vi "Init User Prompt.vi"(0 "Custom Device Ref in":T2 format="%.0x", 11 "error in":errorcluster) -> (3 "Physical Device Name":string, 4 "Temperature Units":T1 items=["Celcius", "Fahrenheit", "Kelvin", "Rankine"], 6 "Dev Chan Count":u32, 8 "High Side Resistor":dbl, 10 "Low Side Resistor":dbl, 15 "error out":errorcluster)   [LabVIEW 2011, in "Simulated Thermocouple Custom Device.lvlib"]
uses:
  Simulated Thermocouple Custom Device.lvlib
  <vilib>/NI Veristand/Custom Device API/Custom Device Item Ref.ctl
  TC Unit Selector.ctl
  Device Settings.ctl
  <vilib>/NI Veristand/Custom Device API/Get Item Property (Variant).vi
  <vilib>/NI Veristand/Custom Device API/Custom Device API.lvlib
panel:
  in  "Device Channel Count":u16(ring)=6 items=["2", "4", "8", "12", "16", "24", "32"]
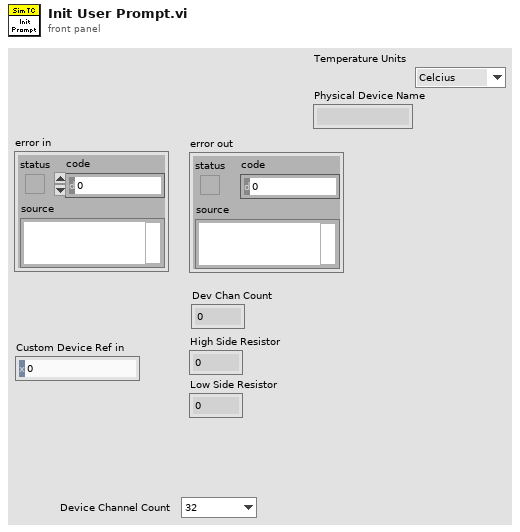
[diagram p1: front panel]
types:
  T1 = typedef "Simulated Thermocouple Custom Device.lvlib/TC Unit Selector.ctl" = u16
  T2 = typedef "Custom Device API.lvlib/Custom Device Item Ref.ctl" = u64
  T3 = typedef "Simulated Thermocouple Custom Device.lvlib/Device Settings.ctl" = cluster{"High Side Resistance (Ohms)":dbl, "Low Side Resistance (Ohms)":dbl, "Temperature Units":T1, "Update Rate":dbl, "Physical Device Name":string, "Device Channel Count":u32}
  T4 = typedef "LVStringsAndValuesArrayTypeDef.ctl" = cluster{"String":string, "Value":u16}[]
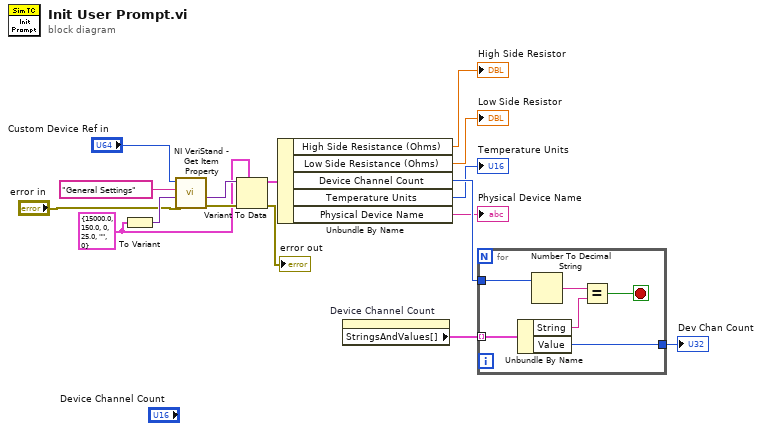
[diagram p0: block diagram]
diagram:
  w6 = T3 {"High Side Resistance (Ohms)"=15000.0, "Low Side Resistance (Ohms)"=150.0, "Temperature Units"=0, "Update Rate"=25.0, "Physical Device Name"="", "Device Channel Count"=0} ("General Settings")
  n1 = To Variant(anything=w6) -> (Variant=w15:variant)
  n2 = call-poly <vilib>:"NI VeriStand - Get Item Property.vi"("error in (no error)"="error in", "Default Value"=w15, "Property Name"="General Settings", "Item Ref in"="Custom Device Ref in") -> ("error out"=w7:errorcluster, "Value"=w8:variant)  [unwired: 4 in, 2 out]
  n3 = Variant To Data(error in=w7, type=w6, Variant=w8) -> (data=w13:T3, error out=→"error out":errorcluster)
  n4 = Unbundle By Name(w13) -> ("High Side Resistance (Ohms)"=→"High Side Resistor":dbl, "Low Side Resistance (Ohms)"=→"Low Side Resistor":dbl, "Device Channel Count"=w5:u32, "Temperature Units"=→"Temperature Units":T1, "Physical Device Name"=→"Physical Device Name":string)
  n5 = property on="Device Channel Count" class="Ring (strict)"() -> ("StringsAndValues[]"=w10:T4)  [unwired: 2 in, 2 out]
  n6 = for {
    tunnel: w10 -> [w22] mode=indexing
    tunnel: [w18] -> w9
    tunnel: w5 -> [w17]
    stop <- w19 stop-if-true
    n7 = Unbundle By Name(w22) -> ("String"=w20:string, "Value"=w18:u16)
    n8 = Number To Decimal String(number=w17) -> (decimal integer string=w21:string)  [unwired: 1 in]
    n9 = Equal?(x=w21, y=w20) -> (x = y?=w19:bool)
  }
  "Dev Chan Count" <- w9
